vi "Configure Multi Eval Meas Limit Inband Emission.vi"(0 "VISA resource name":refnum<visa-resource-name>, 1 "Minimum (-29.2)":dbl=-29.2 format="%^.3e", 2 "RB Power (-57 .0)":dbl=-57.0 format="%^.3e", 3 "IQ Image Greater (-27.2)":dbl=-27.2 format="%^.3e", 5 "Instance (1)":T1=1, 7 "Modulation (Pi/2-BPSK)":i32(ring) items=["Pi/2-BPSK", "Pi/2-BPSK With Shaping", "QPSK", "16-QAM", "64-QAM", "256-QAM"], 9 "Enabled (Off)":bool, 11 "error in (no error)":errorcluster, 12 "EVM (30.0)":dbl=30.0 format="%^.3e", 13 "IQ Image Lesser (-24.2)":dbl=-24.2 format="%^.3e") -> (4 "VISA resource name out":refnum<visa-resource-name>, 15 "error out":errorcluster)   [LabVIEW 2020, in "Rohde&Schwarz CMWXP NR FR1 Measurement.lvlib"]
doc: "Defines parameters used for calculation of an upper limit for the inband emission.\n\nAttributes:\nRSCMWXPNRFR1M_ATTR_MULTI_EVAL_MEAS_LIMIT_PI_2_INBAND_EMISSION\nRSCMWXPNRFR1M_ATTR_MULTI_EVAL_MEAS_LIMIT_BPSK_SHAPING_INBAND_EMISSION\nRSCMWXPNRFR1M_ATTR_MULTI_EVAL_MEAS_LIMIT_QPSK_INBAND_EMISSION\nRSCMWXPNRFR1M_ATTR_MULTI_EVAL_MEAS_LIMIT_QAM_INBAND_EMISSION\n\nRemote-control commands:\nCONFigure:NRSub:MEAS<i>:MEValuation:LIMit:PHBPsk:IBE\nCONFigure:NRSub:MEAS<i>:MEValuation:LIMit:BPWShaping:IBE\nCONFigure:NRSub:MEAS<i>:MEValuation:LIMit:QPSK:IBE\nCONFigure:NRSub:MEAS<i>:MEValuation:LIMit:QAM<order>:IBE"
uses:
  <instrlib>/Rohde&Schwarz CMWXP NR FR1 Measurement/Rohde&Schwarz CMWXP NR FR1 Measurement.lvlib
  <instrlib>/Rohde&Schwarz CMWXP NR FR1 Measurement/Private/_Instance.ctl
  <instrlib>/Rohde&Schwarz CMWXP NR FR1 Measurement/Private/rsidr_core.llb/rsidr_core.lvlib
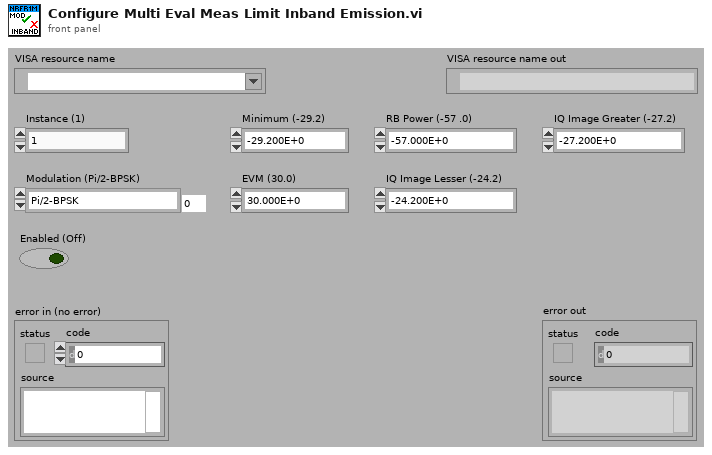
[diagram p1: front panel]
types:
  T1 = typedef "Rohde&Schwarz CMWXP NR FR1 Measurement.lvlib/_Instance.ctl" = i32
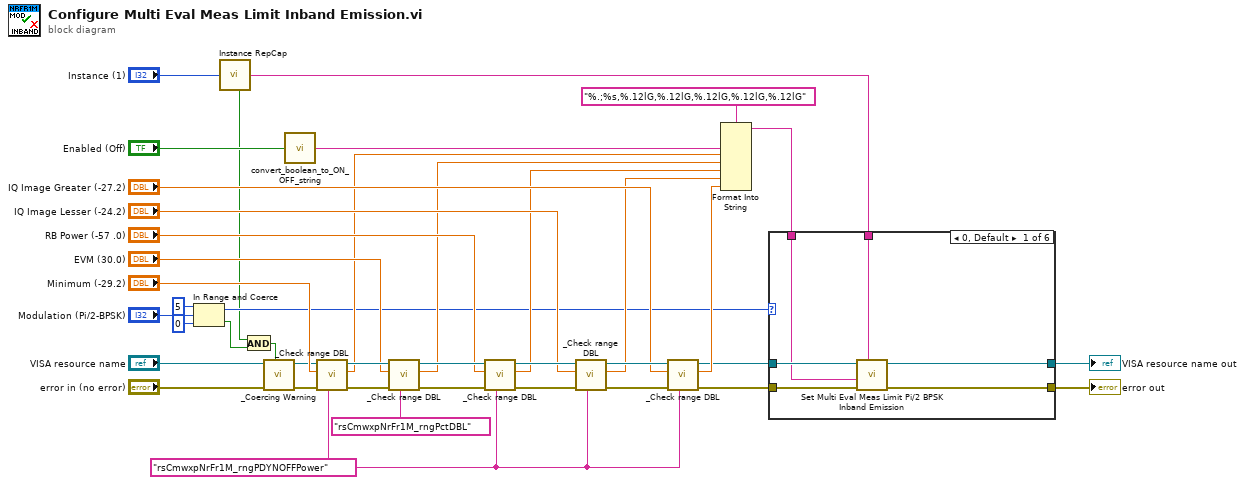
[diagram p0: block diagram]
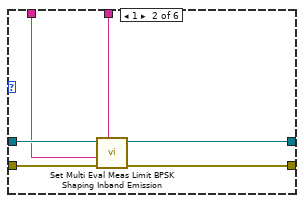
[diagram p2: hidden frame]
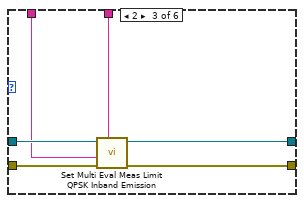
[diagram p3: hidden frame]
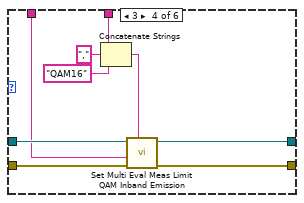
[diagram p4: hidden frame]
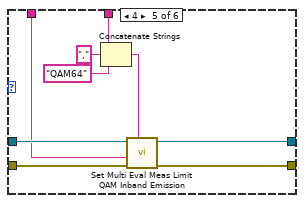
[diagram p5: hidden frame]
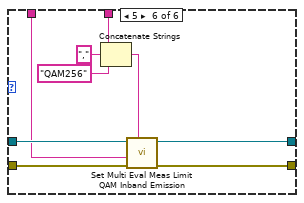
[diagram p6: hidden frame]
diagram:
  w12 = "rsCmwxpNrFr1M_rngPDYNOFFPower" ("Range Table Identifier")
  n1 = In Range and Coerce(upper limit=5, x="Modulation (Pi/2-BPSK)", lower limit=0) -> (coerced(x)=w6:i32, In Range?=w3:bool)
  n2 = call <instrlib>:"Instance RepCap.vi"("Instance In"="Instance (1)") -> ("In Range?"=w1:bool, "RepCap Identifier Out"=w38:string)  [unwired: 1 in]
  n3 = And(x=w1, y=w3) -> (x .and. y?=w2:bool)
  n4 = call <instrlib>:"_Coercing Warning.vi"("In Range?"=w2, "error in (no error)"="error in (no error)", "VISA resource name"="VISA resource name") -> ("error out"=w9:errorcluster, "VISA resource name out"=w8:refnum<visa-resource-name>)  [unwired: 7 in]
  n5 = call <instrlib>:"convert_boolean_to_ON_OFF_string.vi"("boolean value in"="Enabled (Off)") -> ("string value out"=w35:string)  [unwired: 4 in]
  n6 = call <instrlib>:"_Check range DBL.vi"("Range Table Identifier"=w12, "error in (no error)"=w9, "DBL Value In"="Minimum (-29.2)", "VISA resource name"=w8) -> ("error out"=w34:errorcluster, "DBL Value Out"=w21:dbl, "VISA resource name out"=w33:refnum<visa-resource-name>)  [unwired: 5 in]
  n7 = call <instrlib>:"_Check range DBL.vi"("Range Table Identifier"="rsCmwxpNrFr1M_rngPctDBL", "error in (no error)"=w34, "DBL Value In"="EVM (30.0)", "VISA resource name"=w33) -> ("error out"=w32:errorcluster, "DBL Value Out"=w20:dbl, "VISA resource name out"=w31:refnum<visa-resource-name>)  [unwired: 5 in]
  n8 = call <instrlib>:"_Check range DBL.vi"("Range Table Identifier"=w12, "error in (no error)"=w32, "DBL Value In"="RB Power (-57 .0)", "VISA resource name"=w31) -> ("error out"=w30:errorcluster, "DBL Value Out"=w19:dbl, "VISA resource name out"=w29:refnum<visa-resource-name>)  [unwired: 5 in]
  n9 = call <instrlib>:"_Check range DBL.vi"("Range Table Identifier"=w12, "error in (no error)"=w30, "DBL Value In"="IQ Image Lesser (-24.2)", "VISA resource name"=w29) -> ("error out"=w28:errorcluster, "DBL Value Out"=w18:dbl, "VISA resource name out"=w27:refnum<visa-resource-name>)  [unwired: 5 in]
  n10 = call <instrlib>:"_Check range DBL.vi"("Range Table Identifier"=w12, "error in (no error)"=w28, "DBL Value In"="IQ Image Greater (-27.2)", "VISA resource name"=w27) -> ("error out"=w15:errorcluster, "DBL Value Out"=w17:dbl, "VISA resource name out"=w16:refnum<visa-resource-name>)  [unwired: 5 in]
  n11 = Format Into String(format string="%.;%s,%.12lG,%.12lG,%.12lG,%.12lG,%.12lG", w35, w21, w20, w19, w18, w17) -> (resulting string=w14:string)  [unwired: 2 in, 1 out]
  n12 = case shown="0, Default" w6 {
    tunnel: [w47 w53 w59 w68 w77 w86] -> w41
    tunnel: [w46 w52 w58 w67 w76 w85] -> w40
    tunnel: w38 -> [w45 w51 w57 w63 w72 w81]
    tunnel: w16 -> [w44 w50 w56 w66 w75 w84]
    tunnel: w15 -> [w43 w49 w55 w65 w74 w83]
    tunnel: w14 -> [w42 w48 w54 w64 w73 w82]
    frame 0, Default {
      n13 = call "Set Multi Eval Meas Limit Pi/2 BPSK Inband Emission"("Repeated Capabilities"=w45, "error in (no error)"=w43, "Multi Eval Meas Limit Pi/2 BPSK Inband Emission ()"=w42, "instrument handle"=w44) -> ("error out"=w47:errorcluster, "instrument handle out"=w46:refnum<visa-resource-name>)  [unwired: 6 in]
    }
    frame 1 {
      n14 = call "Set Multi Eval Meas Limit BPSK Shaping Inband Emission"("Repeated Capabilities"=w51, "error in (no error)"=w49, "Multi Eval Meas Limit BPSK Shaping Inband Emission ()"=w48, "instrument handle"=w50) -> ("error out"=w53:errorcluster, "instrument handle out"=w52:refnum<visa-resource-name>)  [unwired: 6 in]
    }
    frame 2 {
      n15 = call "Set Multi Eval Meas Limit QPSK Inband Emission"("Repeated Capabilities"=w57, "error in (no error)"=w55, "Multi Eval Meas Limit QPSK Inband Emission ()"=w54, "instrument handle"=w56) -> ("error out"=w59:errorcluster, "instrument handle out"=w58:refnum<visa-resource-name>)  [unwired: 6 in]
    }
    frame 3 {
      n16 = Concatenate Strings(w63, "," ("string"), "QAM16" ("string")) -> (w60:string)
      n17 = call "Set Multi Eval Meas Limit QAM Inband Emission"("Repeated Capabilities"=w60, "error in (no error)"=w65, "Multi Eval Meas Limit QAM Inband Emission ()"=w64, "instrument handle"=w66) -> ("error out"=w68:errorcluster, "instrument handle out"=w67:refnum<visa-resource-name>)  [unwired: 6 in]
    }
    frame 4 {
      n18 = Concatenate Strings(w72, "," ("string"), "QAM64" ("string")) -> (w69:string)
      n19 = call "Set Multi Eval Meas Limit QAM Inband Emission"("Repeated Capabilities"=w69, "error in (no error)"=w74, "Multi Eval Meas Limit QAM Inband Emission ()"=w73, "instrument handle"=w75) -> ("error out"=w77:errorcluster, "instrument handle out"=w76:refnum<visa-resource-name>)  [unwired: 6 in]
    }
    frame 5 {
      n20 = Concatenate Strings(w81, "," ("string"), "QAM256" ("string")) -> (w78:string)
      n21 = call "Set Multi Eval Meas Limit QAM Inband Emission"("Repeated Capabilities"=w78, "error in (no error)"=w83, "Multi Eval Meas Limit QAM Inband Emission ()"=w82, "instrument handle"=w84) -> ("error out"=w86:errorcluster, "instrument handle out"=w85:refnum<visa-resource-name>)  [unwired: 6 in]
    }
  }
  "error out" <- w41
  "VISA resource name out" <- w40
